vi "Clean List of Properties Selection by Type.vi"(11 "Data Cluster in":T1) -> (0 "List of Tags":string[](array[string]), 3 "output cluster":T1)   [LabVIEW 2020, in "Control Property Tree.lvlib"]
uses:
  Control Property Tree.lvlib
  Module Data--cluster.ctl
  Ctrl Properties Map Data.ctl
  Property array.ctl
  Selected Ctrls - List of Controls.ctl
  Selected Ctrls - List of Properties.ctl
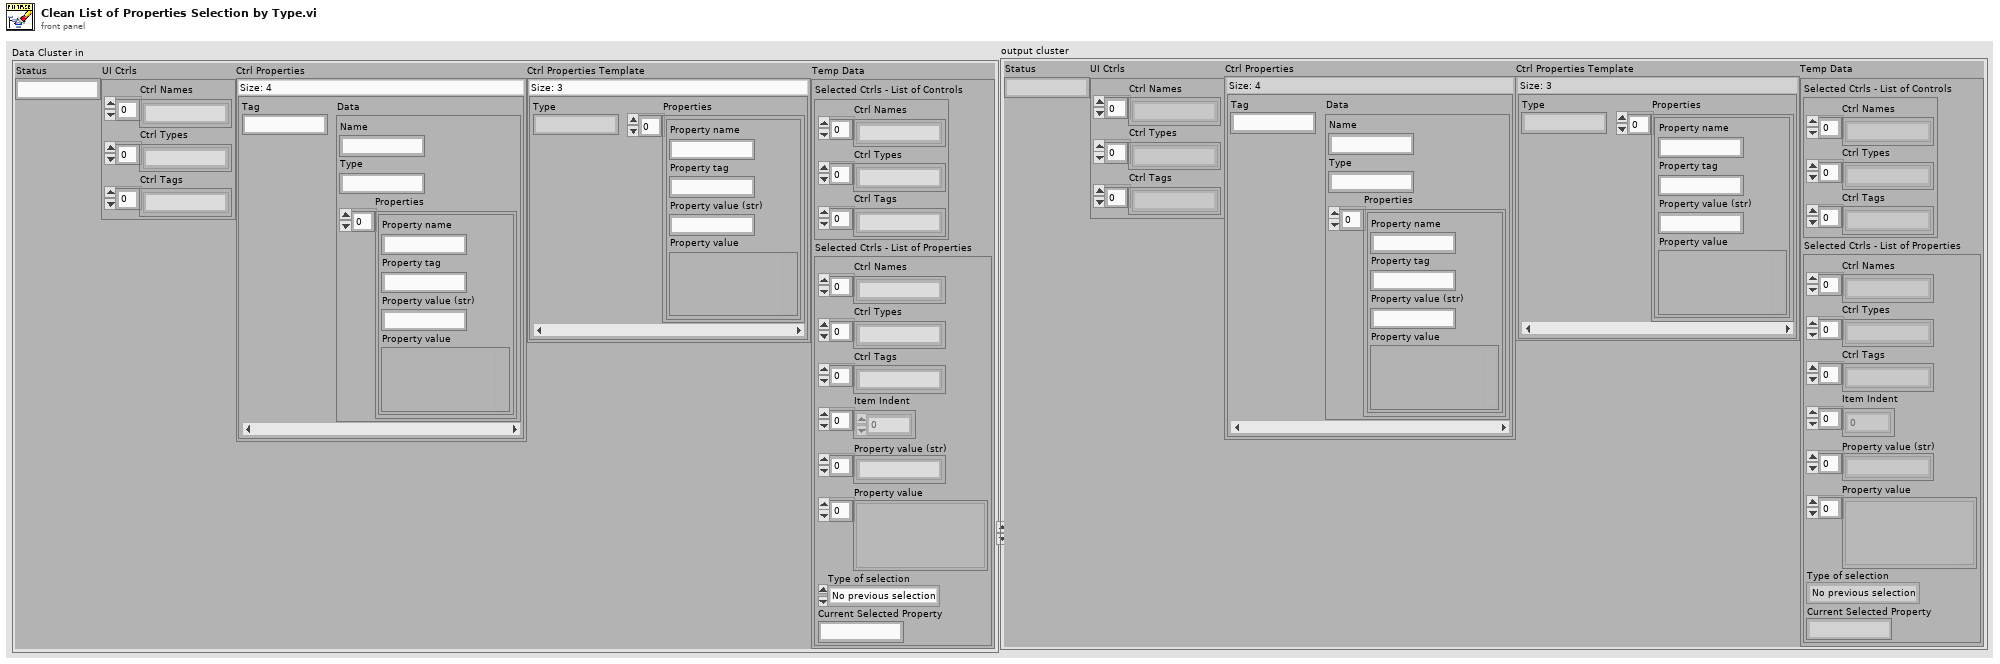
[diagram p1: front panel]
types:
  T1 = typedef "Control Property Tree.lvlib/Module Data--cluster.ctl" = cluster{"Status":string, "UI Ctrls":cluster{"Ctrl Names":string[], "Ctrl Types":string[], "Ctrl Tags":string[]}, "Ctrl Properties":map{string, T2}, "Ctrl Properties Template":map{string, T3}, "Temp Data":cluster{"Selected Ctrls - List of Controls":T4, "Selected Ctrls - List of Properties":T5}}
  T2 = typedef "Control Property Tree.lvlib/Ctrl Properties Map Data.ctl" = cluster{"Name":string, "Type":string, "Properties":T3}
  T3 = typedef "Control Property Tree.lvlib/Property array.ctl" = cluster{"Property name":string, "Property tag":string, "Property value (str)":string, "Property value":variant}[]
  T4 = typedef "Control Property Tree.lvlib/Selected Ctrls - List of Controls.ctl" = cluster{"Ctrl Names":string[], "Ctrl Types":string[], "Ctrl Tags":string[]}
  T5 = typedef "Control Property Tree.lvlib/Selected Ctrls - List of Properties.ctl" = cluster{"Ctrl Names":string[], "Ctrl Types":string[], "Ctrl Tags":string[], "Item Indent":i32[], "Property value (str)":string[], "Property value":variant[], "Type of selection":enum16{"No previous selection", "Control selected", "Property selected"}, "Current Selected Property":string}
  T6 = enum16{"No previous selection", "Control selected", "Property selected"}
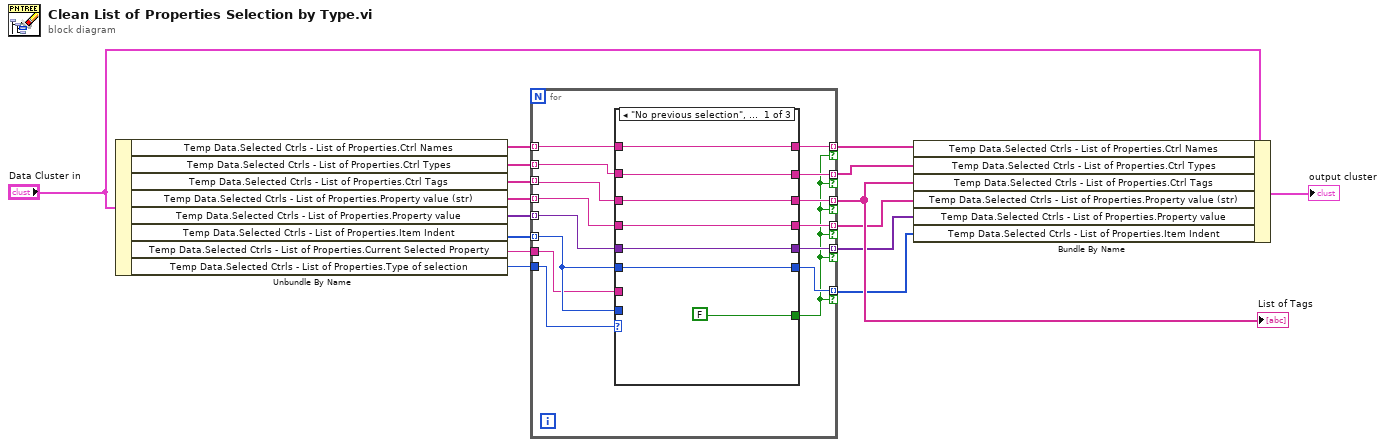
[diagram p0: block diagram]
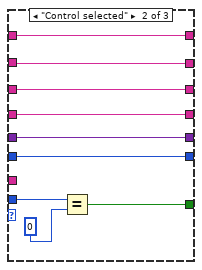
[diagram p2: hidden frame]
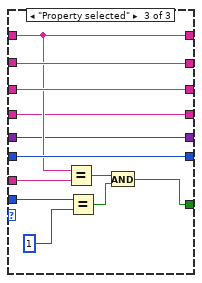
[diagram p3: hidden frame]
diagram:
  n1 = Unbundle By Name("Data Cluster in") -> ("Temp Data.Selected Ctrls - List of Properties.Ctrl Names"=w11:string[], "Temp Data.Selected Ctrls - List of Properties.Ctrl Types"=w10:string[], "Temp Data.Selected Ctrls - List of Properties.Ctrl Tags"=w9:string[], "Temp Data.Selected Ctrls - List of Properties.Property value (str)"=w5:string[], "Temp Data.Selected Ctrls - List of Properties.Property value"=w4:variant[], "Temp Data.Selected Ctrls - List of Properties.Item Indent"=w8:i32[], "Temp Data.Selected Ctrls - List of Properties.Current Selected Property"=w6:string, "Temp Data.Selected Ctrls - List of Properties.Type of selection"=w7:T6)
  n2 = for {
    tunnel: w10 -> [w28] mode=indexing
    tunnel: w11 -> [w29] mode=indexing
    tunnel: w9 -> [w25] mode=indexing
    tunnel: w8 -> [w23] mode=indexing
    tunnel: w7 -> [w31]
    tunnel: [w30] -> w16 mode=indexing if=w17
    tunnel: [w27] -> w15 mode=indexing if=w17
    tunnel: [w26] -> w14 mode=indexing if=w17
    tunnel: [w24] -> w3 mode=indexing if=w17
    tunnel: w6 -> [w22]
    tunnel: w5 -> [w21] mode=indexing
    tunnel: w4 -> [w20] mode=indexing
    tunnel: [w19] -> w2 mode=indexing if=w17
    tunnel: [w18] -> w1 mode=indexing if=w17
    n3 = case shown="\"No previous selection\", Default" w31 {
      tunnel: w23 -> [_ w46 w58]
      tunnel: [FALSE w45 w50] -> w17
      tunnel: [w37 w44 w53] -> w30
      tunnel: w29 -> [w37 w44 w53]
      tunnel: w28 -> [w36 w43 w57]
      tunnel: [w36 w43 w57] -> w27
      tunnel: [w35 w42 w56] -> w26
      tunnel: w25 -> [w35 w42 w56]
      tunnel: [w34 w41 w55] -> w24
      tunnel: w23 -> [w34 w41 w55]
      tunnel: w22 -> [_ _ w54]
      tunnel: w21 -> [w33 w40 w49]
      tunnel: w20 -> [w32 w39 w48]
      tunnel: [w33 w40 w49] -> w19
      tunnel: [w32 w39 w48] -> w18
      frame "No previous selection", Default {
      }
      frame "Control selected" {
        n4 = Equal?(x=w46, y=0) -> (x = y?=w45:bool)
      }
      frame "Property selected" {
        n5 = Equal?(x=w53, y=w54) -> (x = y?=w52:bool)
        n6 = Equal?(x=w58, y=1) -> (x = y?=w51:bool)
        n7 = And(x=w52, y=w51) -> (x .and. y?=w50:bool)
      }
    }
  }
  "List of Tags" <- w14
  n8 = Bundle By Name(cluster="Data Cluster in", "Temp Data.Selected Ctrls - List of Properties.Ctrl Names"=w16, "Temp Data.Selected Ctrls - List of Properties.Ctrl Types"=w15, "Temp Data.Selected Ctrls - List of Properties.Ctrl Tags"=w14, "Temp Data.Selected Ctrls - List of Properties.Property value (str)"=w2, "Temp Data.Selected Ctrls - List of Properties.Property value"=w1, "Temp Data.Selected Ctrls - List of Properties.Item Indent"=w3) -> (→"output cluster":T1)
